vi "Check Date Components.vi"(1 "Input String":string, 2 "Date Type":enum16{"Year", "Month", "Day"}(ring)) -> (0 "Output String":string)   [LabVIEW 2020]
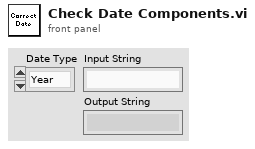
[diagram p1: front panel]
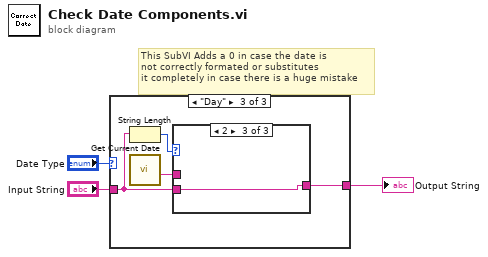
[diagram p0: block diagram]
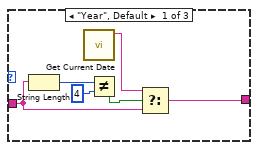
[diagram p2: hidden frame]
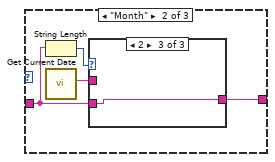
[diagram p3: hidden frame]
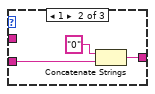
[diagram p5: hidden frame]
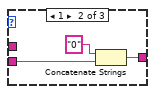
[diagram p7: hidden frame]
diagram:
  # "This SubVI Adds a 0 in case the date is \nnot correctly formated or substitutes \nit completely in case there is a huge mistake"
  n1 = case shown="\"Day\"" "Date Type" {
    tunnel: "Input String" -> [w5 w10 w20]
    tunnel: [w4 w11 w21] -> w1
    frame "Year", Default {
      n2 = String Length(string=w5) -> (length=w9:i32)
      n3 = call "Get Current Date.vi"() -> ("Year"=w6:string)  [unwired: 8 in, 3 out]
      n4 = Not Equal?(x=w9, y=4) -> (x != y?=w7:bool)
      n5 = Select(t=w6, s=w7, f=w5) -> (s? t:f=w4:string)
    }
    frame "Month" {
      n6 = String Length(string=w10) -> (length=w13:i32)
      n7 = call "Get Current Date.vi"() -> ("Month"=w12:string)  [unwired: 8 in, 3 out]
      n8 = case shown="2" w13 {
        tunnel: w12 -> [w14 _ _]
        tunnel: [w14 w15 w18] -> w11
        tunnel: w10 -> [_ w17 w18]
        frame 0, Default {
        }
        frame 1 {
          n9 = Concatenate Strings("0" ("string"), w17) -> (w15:string)
        }
        frame 2 {
        }
      }
    }
    frame "Day" {
      n10 = String Length(string=w20) -> (length=w22:i32)
      n11 = call "Get Current Date.vi"() -> ("Day"=w19:string)  [unwired: 8 in, 3 out]
      n12 = case shown="2" w22 {
        tunnel: w19 -> [w23 _ _]
        tunnel: [w23 w24 w27] -> w21
        tunnel: w20 -> [_ w26 w27]
        frame 0, Default {
        }
        frame 1 {
          n13 = Concatenate Strings("0" ("string"), w26) -> (w24:string)
        }
        frame 2 {
        }
      }
    }
  }
  "Output String" <- w1
